vi "Read from File.vi"(7 "Section Name":string, 8 "error in (no error)":errorcluster, 10 "INI Ref":T1, 11 "Mouse Action in":refnum<class "Mouse Action.lvclass">) -> (0 "error out":errorcluster, 2 "INI Ref out":T1, 3 "Mouse Action out":refnum<class "Mouse Action.lvclass">)   [LabVIEW 2020, in "MacroAssert.lvlib" / "Mouse Action.lvclass"]
doc: "Reads associated parameters from the file identified by <B>INI Ref</B>."
uses:
  Mouse Action.lvclass
  <vilib>/Utility/config.llb/Config Data RefNum.ctl
  Mouse Action Type.ctl
  Button.ctl
  Click Type.ctl
  Relative Movement Type.ctl
  <vilib>/Utility/error.llb/Error Cluster From Error Code.vi
  <vilib>/Utility/config.llb/Read Key (String).vi
  <vilib>/Utility/config.llb/Read Key (I32).vi
  <vilib>/Utility/config.llb/Read Key (Boolean).vi
  Action Step/Action Step.lvclass
  <vilib>/Utility/config.llb/NI_LVConfig.lvlib
  SubVIs/Custom Errors/Custom Errors.lvlib
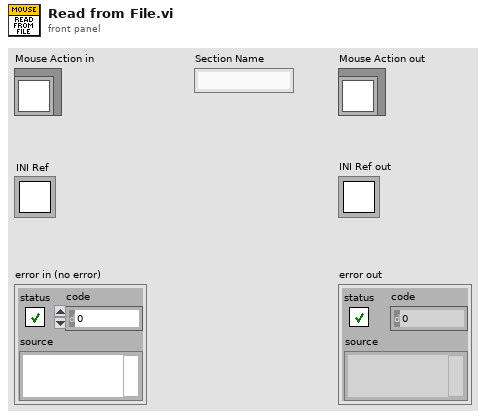
[diagram p1: front panel]
types:
  T1 = typedef "NI_LVConfig.lvlib/Config Data RefNum.ctl" = refnum<k1>
  T2 = typedef "MacroAssert.lvlib/Mouse Action.lvclass/Mouse Action Type.ctl" = enum16{"Click", "Absolute Move", "Absolute Move and Click", "Relative Move", "Relative Move and Click", "Wheel Up", "Wheel Down"}
  T3 = typedef "MacroAssert.lvlib/Mouse Action.lvclass/Button.ctl" = enum16{"Left", "Right", "Middle"}
  T4 = typedef "MacroAssert.lvlib/Mouse Action.lvclass/Click Type.ctl" = enum16{"Normal", "Hold", "Release"}
  T5 = typedef "MacroAssert.lvlib/Mouse Action.lvclass/Relative Movement Type.ctl" = enum16{"Pixels from Current Position", "Pixels from Top-Left of Control", "Pixels from Top-Left of Window", "Percentage from Top-Left of Control", "Percentage from Top-Left of Window", "Percentage from Top-Left of Screen"}
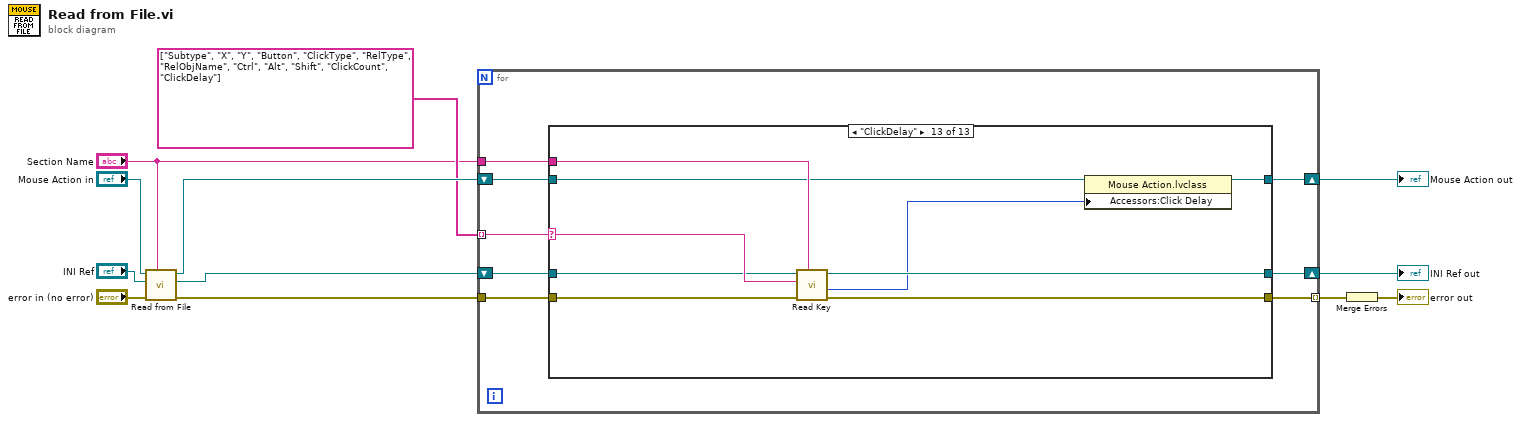
[diagram p0: block diagram]
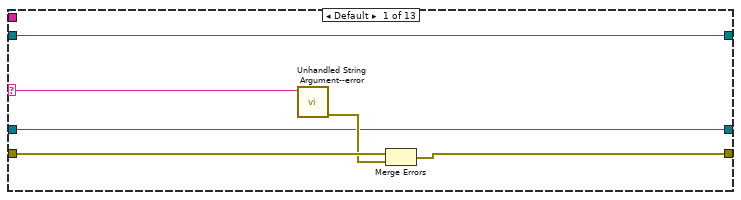
[diagram p2: hidden frame]
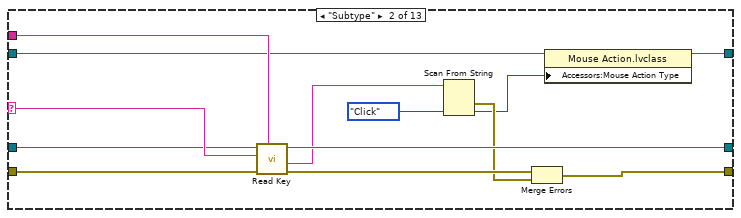
[diagram p3: hidden frame]
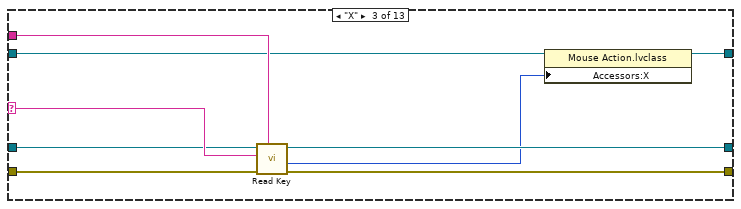
[diagram p4: hidden frame]
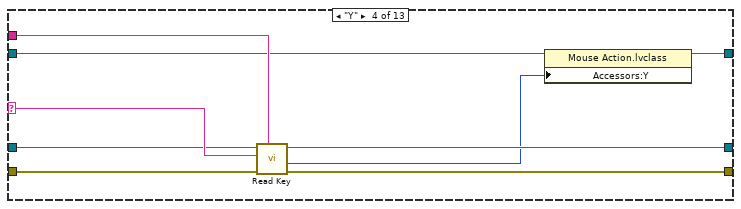
[diagram p5: hidden frame]
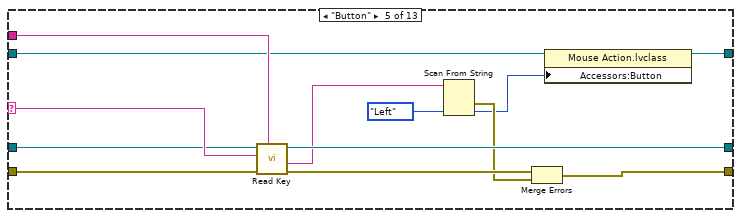
[diagram p6: hidden frame]
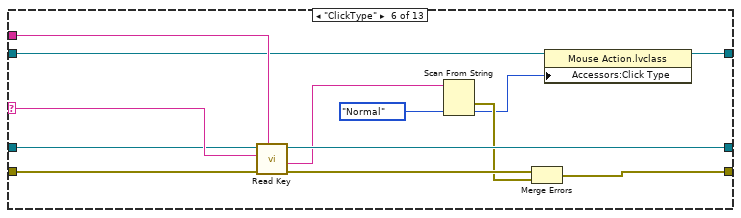
[diagram p7: hidden frame]
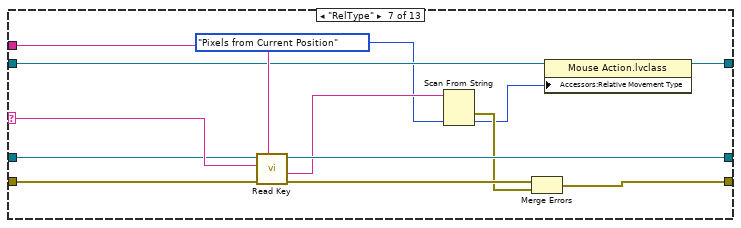
[diagram p8: hidden frame]
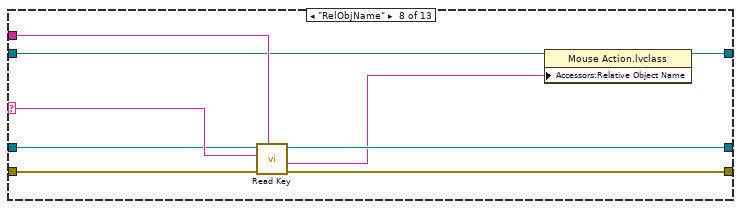
[diagram p9: hidden frame]
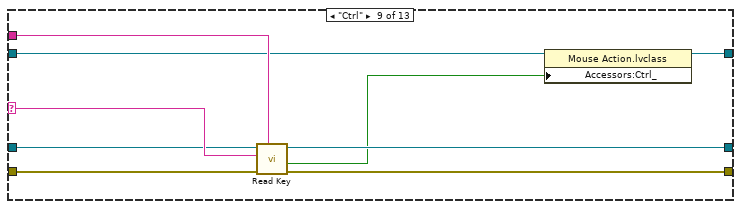
[diagram p10: hidden frame]
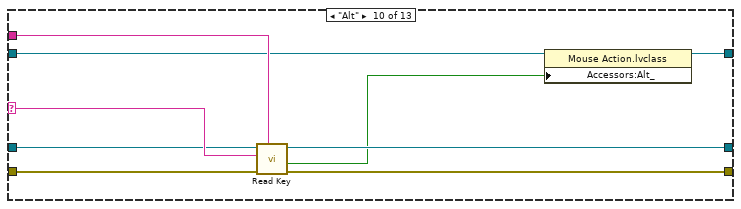
[diagram p11: hidden frame]
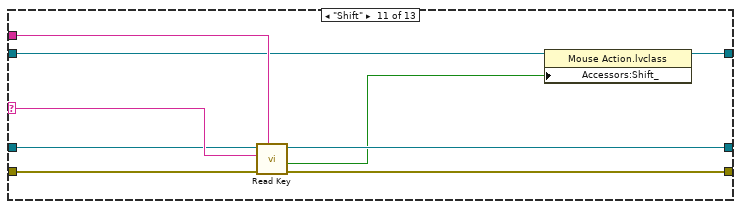
[diagram p12: hidden frame]
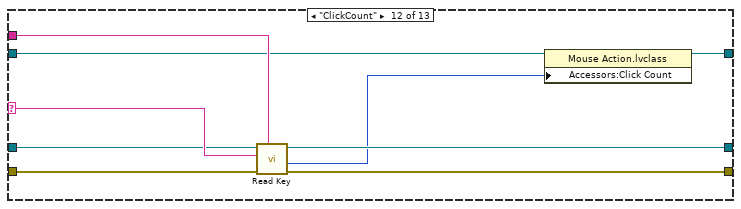
[diagram p13: hidden frame]
diagram:
  n1 = call-parent "Read from File.vi"("Section Name"="Section Name", "error in (no error)"="error in (no error)", "INI Ref"="INI Ref", "Step in"="Mouse Action in") -> ("error out"=w7:errorcluster, "INI Ref out"=w6:T1, "Step out"=w9:refnum<class "Mouse Action.lvclass">)  [unwired: 5 in]
  n2 = for {
    tunnel: string[] ["Subtype", "X", "Y", "Button", "ClickType", "RelType", "RelObjName", "Ctrl", "Alt", "Shift", "ClickCount", "ClickDelay"] -> [w20] mode=indexing
    tunnel: w7 -> [w19]
    tunnel: "Section Name" -> [w18]
    shift-right: [w16] -> w5
    shift-left: w9 -> [w17]
    tunnel: [w15] -> w4 mode=indexing
    shift-right: [w13] -> w2
    shift-left: w6 -> [w14]
    n3 = case shown="\"ClickDelay\"" w20 {
      selector: w20 -> [w23 w34 w43 w52 w65 w78 w91 w100 w109 w118 w127 w136 w145]
      tunnel: w19 -> [w25 w39 w48 w57 w70 w83 w96 w105 w114 w123 w132 w141 w150]
      tunnel: w18 -> [_ w38 w47 w56 w69 w82 w95 w104 w113 w122 w131 w140 w149]
      tunnel: w17 -> [w26 w37 w46 w55 w68 w81 w94 w103 w112 w121 w130 w139 w148]
      tunnel: [w26 w36 w45 w54 w67 w80 w93 w102 w111 w120 w129 w138 w147] -> w16
      tunnel: [w22 w30 w44 w53 w60 w74 w87 w101 w110 w119 w128 w137 w146] -> w15
      tunnel: w14 -> [w21 w33 w42 w51 w64 w77 w90 w99 w108 w117 w126 w135 w144]
      tunnel: [w21 w32 w41 w50 w63 w76 w89 w98 w107 w116 w125 w134 w143] -> w13
      frame Default {
        n4 = call "Unhandled String Argument--error.vi"("Argument"=w23) -> ("error out"=w24:errorcluster)  [unwired: 10 in]
        n5 = Merge Errors(w25, w24) -> (w22:errorcluster)
      }
      frame "Subtype" {
        n6 = call-poly <vilib>:"Read Key.vi"("section"=w38, "error in (no error)"=w39, "key"=w34, "refnum"=w33) -> ("error out"=w35:errorcluster, "value"=w31:string, "refnum out"=w32:T1)  [unwired: 4 in, 1 out]
        n7 = Scan From String(input string=w31, default 1=Mouse_Action_Type."Click" ("Mouse Action Type")) -> (error out=w29:errorcluster, output 1=w28:T2)  [unwired: 3 in, 2 out]
        n8 = Merge Errors(w35, w29) -> (w30:errorcluster)
        n9 = property class="Mouse Action.lvclass"(reference=w37, "Accessors:Mouse Action Type"=w28) -> (reference out=w36:refnum<class "Mouse Action.lvclass">)  [unwired: 1 in, 1 out]
      }
      frame "X" {
        n10 = call-poly <vilib>:"Read Key.vi"("section"=w47, "error in (no error)"=w48, "key"=w43, "refnum"=w42) -> ("error out"=w44:errorcluster, "value"=w40:i32, "refnum out"=w41:T1)  [unwired: 4 in, 1 out]
        n11 = property class="Mouse Action.lvclass"(reference=w46, "Accessors:X"=w40) -> (reference out=w45:refnum<class "Mouse Action.lvclass">)  [unwired: 1 in, 1 out]
      }
      frame "Y" {
        n12 = call-poly <vilib>:"Read Key.vi"("section"=w56, "error in (no error)"=w57, "key"=w52, "refnum"=w51) -> ("error out"=w53:errorcluster, "value"=w49:i32, "refnum out"=w50:T1)  [unwired: 4 in, 1 out]
        n13 = property class="Mouse Action.lvclass"(reference=w55, "Accessors:Y"=w49) -> (reference out=w54:refnum<class "Mouse Action.lvclass">)  [unwired: 1 in, 1 out]
      }
      frame "Button" {
        n14 = call-poly <vilib>:"Read Key.vi"("section"=w69, "error in (no error)"=w70, "key"=w65, "refnum"=w64) -> ("error out"=w66:errorcluster, "value"=w61:string, "refnum out"=w63:T1)  [unwired: 4 in, 1 out]
        n15 = Scan From String(input string=w61, default 1=Button."Left" ("Button")) -> (error out=w59:errorcluster, output 1=w58:T3)  [unwired: 3 in, 2 out]
        n16 = Merge Errors(w66, w59) -> (w60:errorcluster)
        n17 = property class="Mouse Action.lvclass"(reference=w68, "Accessors:Button"=w58) -> (reference out=w67:refnum<class "Mouse Action.lvclass">)  [unwired: 1 in, 1 out]
      }
      frame "ClickType" {
        n18 = call-poly <vilib>:"Read Key.vi"("section"=w82, "error in (no error)"=w83, "key"=w78, "refnum"=w77) -> ("error out"=w79:errorcluster, "value"=w75:string, "refnum out"=w76:T1)  [unwired: 4 in, 1 out]
        n19 = Scan From String(input string=w75, default 1=Click_Type."Normal" ("Click Type")) -> (error out=w73:errorcluster, output 1=w72:T4)  [unwired: 3 in, 2 out]
        n20 = Merge Errors(w79, w73) -> (w74:errorcluster)
        n21 = property class="Mouse Action.lvclass"(reference=w81, "Accessors:Click Type"=w72) -> (reference out=w80:refnum<class "Mouse Action.lvclass">)  [unwired: 1 in, 1 out]
      }
      frame "RelType" {
        n22 = call-poly <vilib>:"Read Key.vi"("section"=w95, "error in (no error)"=w96, "key"=w91, "refnum"=w90) -> ("error out"=w92:errorcluster, "value"=w88:string, "refnum out"=w89:T1)  [unwired: 4 in, 1 out]
        n23 = Scan From String(input string=w88, default 1=Relative_Movement_Type."Pixels from Current Position" ("Relative Movement Type")) -> (error out=w86:errorcluster, output 1=w85:T5)  [unwired: 3 in, 2 out]
        n24 = Merge Errors(w92, w86) -> (w87:errorcluster)
        n25 = property class="Mouse Action.lvclass"(reference=w94, "Accessors:Relative Movement Type"=w85) -> (reference out=w93:refnum<class "Mouse Action.lvclass">)  [unwired: 1 in, 1 out]
      }
      frame "RelObjName" {
        n26 = call-poly <vilib>:"Read Key.vi"("section"=w104, "error in (no error)"=w105, "key"=w100, "refnum"=w99) -> ("error out"=w101:errorcluster, "value"=w97:string, "refnum out"=w98:T1)  [unwired: 4 in, 1 out]
        n27 = property class="Mouse Action.lvclass"(reference=w103, "Accessors:Relative Object Name"=w97) -> (reference out=w102:refnum<class "Mouse Action.lvclass">)  [unwired: 1 in, 1 out]
      }
      frame "Ctrl" {
        n28 = call-poly <vilib>:"Read Key.vi"("section"=w113, "error in (no error)"=w114, "key"=w109, "refnum"=w108) -> ("error out"=w110:errorcluster, "value"=w106:bool, "refnum out"=w107:T1)  [unwired: 4 in, 1 out]
        n29 = property class="Mouse Action.lvclass"(reference=w112, "Accessors:Ctrl_"=w106) -> (reference out=w111:refnum<class "Mouse Action.lvclass">)  [unwired: 1 in, 1 out]
      }
      frame "Alt" {
        n30 = call-poly <vilib>:"Read Key.vi"("section"=w122, "error in (no error)"=w123, "key"=w118, "refnum"=w117) -> ("error out"=w119:errorcluster, "value"=w115:bool, "refnum out"=w116:T1)  [unwired: 4 in, 1 out]
        n31 = property class="Mouse Action.lvclass"(reference=w121, "Accessors:Alt_"=w115) -> (reference out=w120:refnum<class "Mouse Action.lvclass">)  [unwired: 1 in, 1 out]
      }
      frame "Shift" {
        n32 = call-poly <vilib>:"Read Key.vi"("section"=w131, "error in (no error)"=w132, "key"=w127, "refnum"=w126) -> ("error out"=w128:errorcluster, "value"=w124:bool, "refnum out"=w125:T1)  [unwired: 4 in, 1 out]
        n33 = property class="Mouse Action.lvclass"(reference=w130, "Accessors:Shift_"=w124) -> (reference out=w129:refnum<class "Mouse Action.lvclass">)  [unwired: 1 in, 1 out]
      }
      frame "ClickCount" {
        n34 = call-poly <vilib>:"Read Key.vi"("section"=w140, "error in (no error)"=w141, "key"=w136, "refnum"=w135) -> ("error out"=w137:errorcluster, "value"=w133:i32, "refnum out"=w134:T1)  [unwired: 4 in, 1 out]
        n35 = property class="Mouse Action.lvclass"(reference=w139, "Accessors:Click Count"=w133) -> (reference out=w138:refnum<class "Mouse Action.lvclass">)  [unwired: 1 in, 1 out]
      }
      frame "ClickDelay" {
        n36 = call-poly <vilib>:"Read Key.vi"("section"=w149, "error in (no error)"=w150, "key"=w145, "refnum"=w144) -> ("error out"=w146:errorcluster, "value"=w142:i32, "refnum out"=w143:T1)  [unwired: 4 in, 1 out]
        n37 = property class="Mouse Action.lvclass"(reference=w148, "Accessors:Click Delay"=w142) -> (reference out=w147:refnum<class "Mouse Action.lvclass">)  [unwired: 1 in, 1 out]
      }
    }
  }
  "Mouse Action out" <- w5
  "INI Ref out" <- w2
  n38 = Merge Errors(w4) -> (→"error out":errorcluster)
